vi "Reset.vi"(8 "error in (no error)":errorcluster, 10 "Message in":refnum<class "ResetMessage.lvclass">=refnum, 11 "PockelCell in":refnum<class "PockelCell.lvclass">) -> (0 "error out":errorcluster, 3 "PockelCell out":refnum<class "PockelCell.lvclass">)   [LabVIEW 2012, in "PockelCell.lvclass"]
doc: "The reset method processes the command 'reset'. \n\nResets the internal state of the component (without performing a full initialisation). This could be resetting hardware, or private data to default values."
uses:
  PockelCell.lvclass
  Murmex/LabVIEW/Murmex/StopMessage/StopMessage.lvclass
  Murmex/LabVIEW/Murmex/StartMessage/StartMessage.lvclass
  <vilib>/Distrio/Murmex/Murmex/Murmex.lvclass
  Murmex/LabVIEW/Murmex/ResetMessage/ResetMessage.lvclass
panel:
  # "This method is called when the RESET\ntrigger is sent. \n\nOverride this method when your component needs to\nrespond to this trigger. \n\nCall parent for proper implementation"
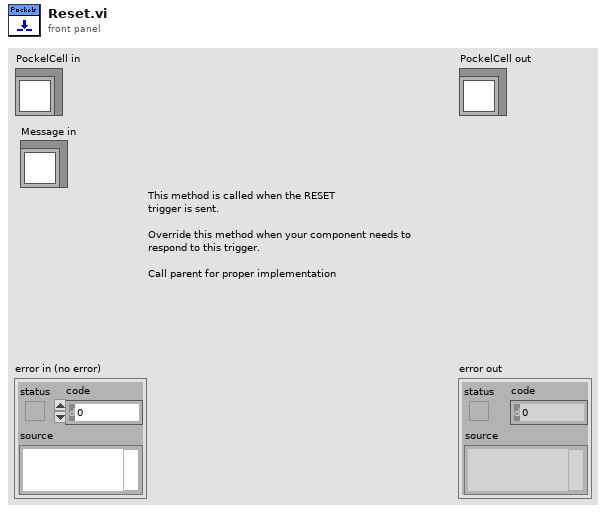
[diagram p1: front panel]
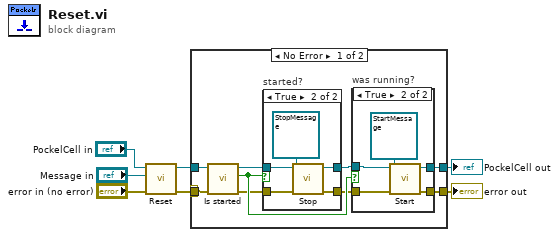
[diagram p0: block diagram]
diagram:
  n1 = call-parent "Reset.vi"("error in (no error)"="error in (no error)", "Message in"="Message in", "Murmex in"="PockelCell in") -> ("error out"=w3:errorcluster, "Murmex out"=w4:refnum<class "PockelCell.lvclass">)  [unwired: 7 in]
  n2 = case shown="No Error" w3 {
    selector: w3 -> [_ w31]
    tunnel: w3 -> [w16 _]
    tunnel: w4 -> [w15 w32]
    tunnel: [w9 w31] -> w2
    tunnel: [w8 w32] -> w1
    frame No Error {
      n3 = call "Is started.vi"("error in (no error)"=w16, "Murmex in"=w15) -> ("error out"=w13:errorcluster, "started?"=w14:bool, "Murmex out"=w12:refnum<class "PockelCell.lvclass">)  [unwired: 7 in]
      n4 = case "started?" shown="True" w14 {
        tunnel: w13 -> [w24 w30]
        tunnel: w12 -> [w25 w28]
        tunnel: [w25 w27] -> w11
        tunnel: [w24 w26] -> w10
        frame False {
        }
        frame True {
          n5 = call-dynamic "Stop.vi"("error in (no error)"=w30, "Message in"=refnum<class "StopMessage.lvclass"> refnum ("StopMessage"), "PockelCell in"=w28) -> ("error out"=w26:errorcluster, "PockelCell out"=w27:refnum<class "PockelCell.lvclass">)  [unwired: 7 in]
        }
      }
      n6 = case "was running?" shown="True" w14 {
        tunnel: w11 -> [w18 w23]
        tunnel: w10 -> [w17 w22]
        tunnel: [w17 w21] -> w9
        tunnel: [w18 w20] -> w8
        frame False {
        }
        frame True {
          n7 = call-dynamic "Start.vi"("error in (no error)"=w22, "Message in"=refnum<class "StartMessage.lvclass"> refnum ("StartMessage"), "PockelCell in"=w23) -> ("error out"=w21:errorcluster, "PockelCell out"=w20:refnum<class "PockelCell.lvclass">)  [unwired: 7 in]
        }
      }
    }
    frame Error {
    }
  }
  "error out" <- w2
  "PockelCell out" <- w1
